vi "Constants.vi"() -> ()   [LabVIEW 2015, in "Test Shared.lvlib"]
doc: "Use this Global VI to access the GUIDs assigned to the page resources of the Custom Device."
uses:
  Test Shared.lvlib
panel:
  in  "Tab Control":enum32{"GUIDS", "Constants", "Properties"}(tab)
  in  "Test":string="7b2910d9-26d1-4fc0-85f8-778002f60e93"
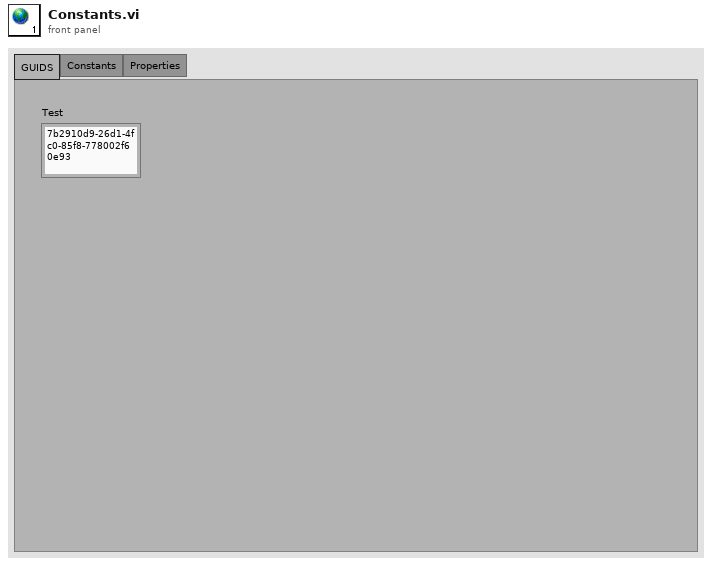
[diagram p1: front panel]
diagram:
